vi "Read MGLT.vi"(8 "error in (no error)":errorcluster, 11 "Hyperspace_SpaceShip in":refnum<class "Hyperspace_SpaceShip.lvclass">) -> (0 "error out":errorcluster, 2 "MGLT":dbl, 3 "Hyperspace_SpaceShip out":refnum<class "Hyperspace_SpaceShip.lvclass">)   [LabVIEW 2021, in "Hyperspace_SpaceShip.lvclass"]
uses:
  Hyperspace_SpaceShip.lvclass
  Hyperspace_SpaceShip.lvclass/Hyperspace_SpaceShip.ctl
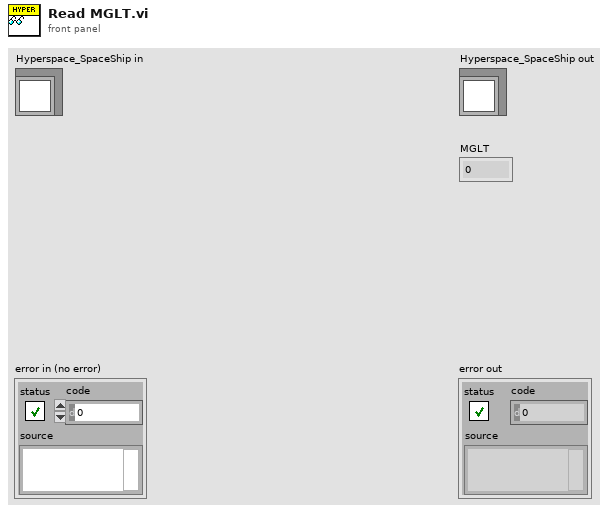
[diagram p1: front panel]
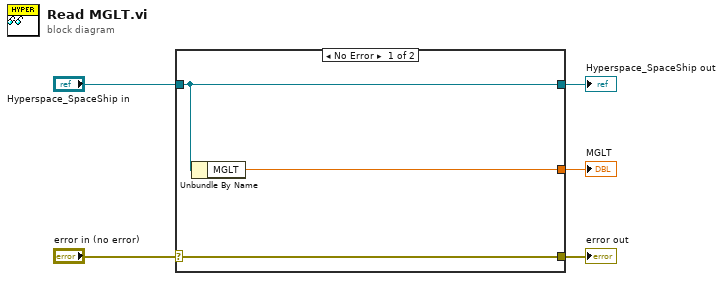
[diagram p0: block diagram]
diagram:
  n1 = case shown="No Error" "error in (no error)" {
    selector: "error in (no error)" -> [w8 w9]
    tunnel: [w8 w9] -> w4
    tunnel: [w7 w10] -> w2
    tunnel: "Hyperspace_SpaceShip in" -> [w7 w10]
    tunnel: [w6 _] -> w1
    frame No Error {
      n2 = Unbundle By Name(w7) -> ("MGLT"=w6:dbl)
    }
    frame Error {
    }
  }
  "error out" <- w4
  "Hyperspace_SpaceShip out" <- w2
  "MGLT" <- w1
